vi "Send Single TCP-IP Cmd Abort.vi"(0 "TCP/IP ID":refnum<k5>, 1 "Buffer/Avg #/Frames":u16, 2 "Mode":u16, 3 "Exposure Time (ms)":u32, 4 "Camera Color":string(combo), 5 "Error In":errorcluster, 6 "Function #":u16, 7 "File Name":string, 9 "Parameter Value":i32, 10 "Camera ID":u8=1, 11 "Save As":u16(ring) items=["U16 FITS", "I16 FITS", "I32 FITS", "SGL FITS", "U16 TIFF", "I16 TIFF", "I32 TIFF", "SGL TIFF"], 12 "Acq. Mode/Type/Frame Mode/RO Mode #":u8, 13 "CCD Format Parameters":T1={"Serial Origin"=50, "Serial Length"=512, "Serial Binning"=1, "Parallel Origin"=0, "Parallel Length"=1024, "Parallel Binning"=1} {"Parallel Binning" min=1 max=5000 step=1; "Parallel Length" min=0 max=65535 step=1; "Parallel Origin" min=0 max=9000 step=1; "Serial Binning" min=1 max=5000 step=1; "Serial Length" min=0 max=65535 step=1; "Serial Origin" min=0 max=9000 step=1}) -> (14 "TCP/IP ID Out":refnum<k5>, 15 "Cmd Packet":string, 17 "Data Type":i32, 18 "Packet ID":i32, 19 "Error Out":errorcluster)   [LabVIEW 2015]
uses:
  Systems/SIcamera_Control/SI_Client_Subvis/CCD Format.ctl
panel:
  # "Parallel"
  # "Serial"
  # "Origin"
  # "Length"
  # "Binning"
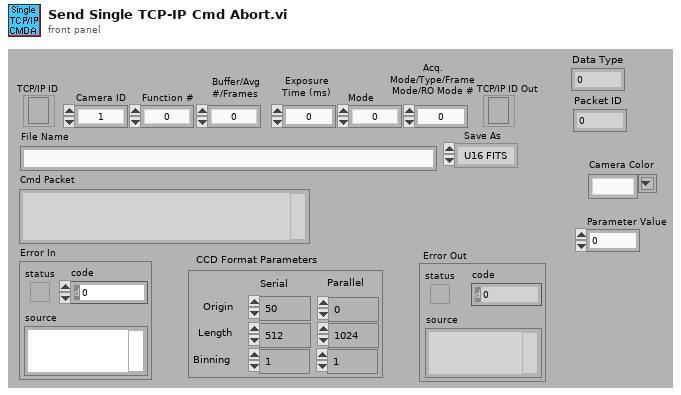
[diagram p1: front panel]
types:
  T1 = typedef "CCD Format.ctl" = cluster{"Serial Origin":i32, "Serial Length":i32, "Serial Binning":i32, "Parallel Origin":i32, "Parallel Length":i32, "Parallel Binning":i32}
  T2 = cluster{"% Exp.":u16, "%Readout":u16, "Relative Pos.":u32, "Acquiring":i32}
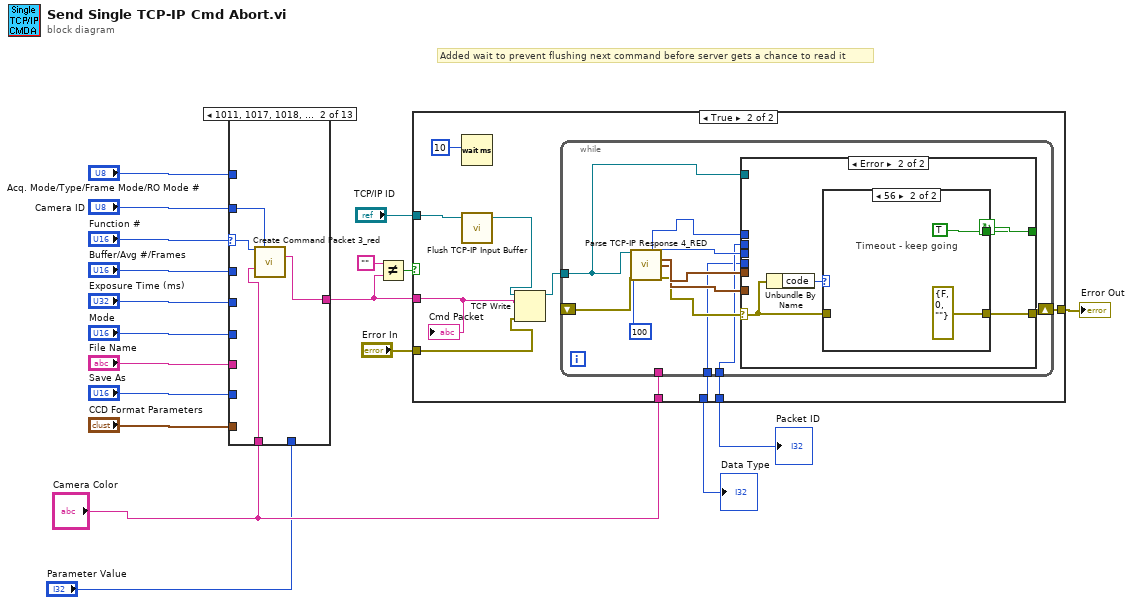
[diagram p0: block diagram]
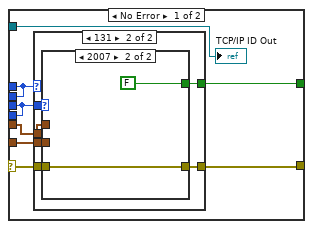
[diagram p3: hidden frame]
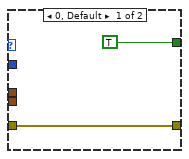
[diagram p4: hidden frame]
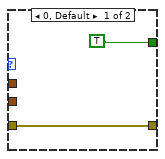
[diagram p5: hidden frame]
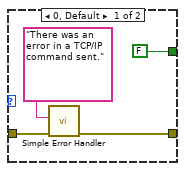
[diagram p6: hidden frame]
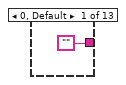
[diagram p7: hidden frame]
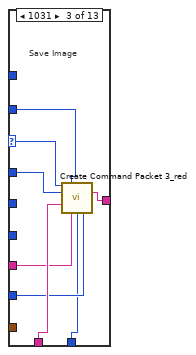
[diagram p8: hidden frame]
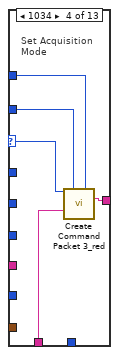
[diagram p9: hidden frame]
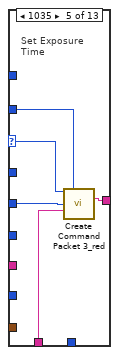
[diagram p10: hidden frame]
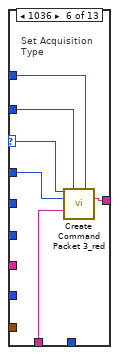
[diagram p11: hidden frame]
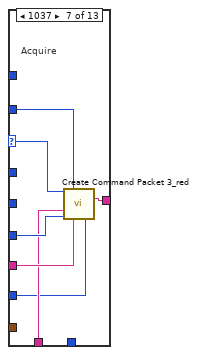
[diagram p12: hidden frame]
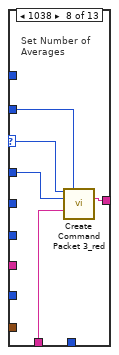
[diagram p13: hidden frame]
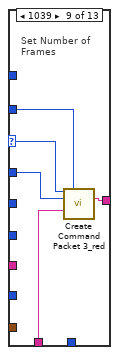
[diagram p14: hidden frame]
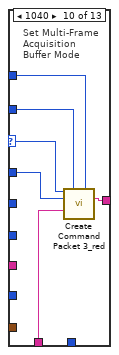
[diagram p15: hidden frame]
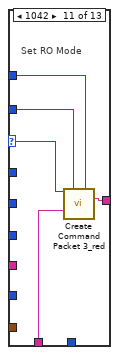
[diagram p16: hidden frame]
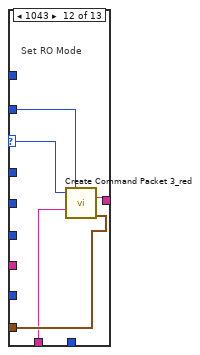
[diagram p17: hidden frame]
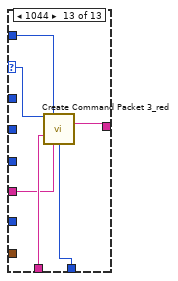
[diagram p18: hidden frame]
diagram:
  # "Added wait to prevent flushing next command before server gets a chance to read it"
  n1 = case shown="1011, 1017, 1018, 1041" "Function #" {
    selector: "Function #" -> [_ w22 w30 w35 w40 w46 w53 w58 w63 w69 w74 w80 w82]
    tunnel: ["" w24 w26 w37 w42 w48 w55 w60 w65 w71 w76 w81 w87] -> w10
    tunnel: "Acq. Mode/Type/Frame Mode/RO Mode #" -> [_ _ _ w34 _ w45 _ _ _ w67 w73 _ _]
    tunnel: "Camera ID" -> [_ w23 w31 w36 w41 w47 w54 w59 w64 w70 w75 w79 w83]
    tunnel: "Buffer/Avg #/Frames" -> [_ _ w29 _ _ w44 _ w57 w62 w68 _ _ _]
    tunnel: "Exposure Time (ms)" -> [_ _ _ _ w39 _ _ _ _ _ _ _ _]
    tunnel: "Mode" -> [_ _ _ _ _ _ w51 _ _ _ _ _ _]
    tunnel: "File Name" -> [_ _ w28 _ _ _ w52 _ _ _ _ _ w84]
    tunnel: "Save As" -> [_ _ w27 _ _ _ w49 _ _ _ _ _ _]
    tunnel: "CCD Format Parameters" -> [_ _ _ _ _ _ _ _ _ _ _ w78 _]
    tunnel: "Camera Color" -> [_ w21 w32 w33 w38 w43 w50 w56 w61 w66 w72 w77 w86]
    tunnel: "Parameter Value" -> [_ _ w25 _ _ _ _ _ _ _ _ _ w85]
    frame 0, Default {
    }
    frame 1011, 1017, 1018, 1041 {
      n2 = call "Create Command Packet 3_red.vi"("Function #"=w22, "Camera ID (1)"=w23, "Camera Color"=w21) -> ("Cmd Packet"=w24:string)  [unwired: 12 in]
    }
    frame 1031 {
      # "Save Image"
      n3 = call "Create Command Packet 3_red.vi"("Function #"=w30, "Camera ID (1)"=w31, "Buffer/Avg #/Frames"=w29, "Camera Color"=w32, "File Name"=w28, "Paramater value"=w25, "Save As"=w27) -> ("Cmd Packet"=w26:string)  [unwired: 8 in]
    }
    frame 1034 {
      # "Set Acquisition Mode"
      n4 = call "Create Command Packet 3_red.vi"("Function #"=w35, "Camera ID (1)"=w36, "Acq. Mode/Type/Frame Mode/RO Mode"=w34, "Camera Color"=w33) -> ("Cmd Packet"=w37:string)  [unwired: 11 in]
    }
    frame 1035 {
      # "Set Exposure Time"
      n5 = call "Create Command Packet 3_red.vi"("Function #"=w40, "Camera ID (1)"=w41, "Exposure Time (ms)"=w39, "Camera Color"=w38) -> ("Cmd Packet"=w42:string)  [unwired: 11 in]
    }
    frame 1036 {
      # "Set Acquisition Type"
      n6 = call "Create Command Packet 3_red.vi"("Function #"=w46, "Camera ID (1)"=w47, "Acq. Mode/Type/Frame Mode/RO Mode"=w45, "Buffer/Avg #/Frames"=w44, "Camera Color"=w43) -> ("Cmd Packet"=w48:string)  [unwired: 10 in]
    }
    frame 1037 {
      # "Acquire"
      n7 = call "Create Command Packet 3_red.vi"("Function #"=w53, "Camera ID (1)"=w54, "Camera Color"=w50, "Mode"=w51, "File Name"=w52, "Save As"=w49) -> ("Cmd Packet"=w55:string)  [unwired: 9 in]
    }
    frame 1038 {
      # "Set Number of Averages"
      n8 = call "Create Command Packet 3_red.vi"("Function #"=w58, "Camera ID (1)"=w59, "Buffer/Avg #/Frames"=w57, "Camera Color"=w56) -> ("Cmd Packet"=w60:string)  [unwired: 11 in]
    }
    frame 1039 {
      # "Set Number of Frames"
      n9 = call "Create Command Packet 3_red.vi"("Function #"=w63, "Camera ID (1)"=w64, "Buffer/Avg #/Frames"=w62, "Camera Color"=w61) -> ("Cmd Packet"=w65:string)  [unwired: 11 in]
    }
    frame 1040 {
      # "Set Multi-Frame Acquisition Buffer Mode"
      n10 = call "Create Command Packet 3_red.vi"("Function #"=w69, "Camera ID (1)"=w70, "Acq. Mode/Type/Frame Mode/RO Mode"=w67, "Buffer/Avg #/Frames"=w68, "Camera Color"=w66) -> ("Cmd Packet"=w71:string)  [unwired: 10 in]
    }
    frame 1042 {
      # "Set RO Mode"
      n11 = call "Create Command Packet 3_red.vi"("Function #"=w74, "Camera ID (1)"=w75, "Acq. Mode/Type/Frame Mode/RO Mode"=w73, "Camera Color"=w72) -> ("Cmd Packet"=w76:string)  [unwired: 11 in]
    }
    frame 1043 {
      # "Set RO Mode"
      n12 = call "Create Command Packet 3_red.vi"("Function #"=w80, "Camera ID (1)"=w79, "Camera Color"=w77, "CCD Format Parameters"=w78) -> ("Cmd Packet"=w81:string)  [unwired: 11 in]
    }
    frame 1044 {
      n13 = call "Create Command Packet 3_red.vi"("Function #"=w82, "Camera ID (1)"=w83, "Camera Color"=w86, "File Name"=w84, "Paramater value"=w85) -> ("Cmd Packet"=w87:string)  [unwired: 10 in]
    }
  }
  n14 = Not Equal?(x="", y=w10) -> (x != y?=w11:bool)
  n15 = case shown="True" w11 {
    tunnel: w10 -> [_ w93]
    tunnel: "TCP/IP ID" -> [_ w98]
    tunnel: "Error In" -> [w88 w94]
    tunnel: [w88 w97] -> w7
    tunnel: "Camera Color" -> [_ w96]
    tunnel: [_ w90] -> w2
    tunnel: [_ w89] -> w1
    frame False {
    }
    frame True {
      n16 = Wait (ms)(milliseconds to wait=u32 10) -> ()  [unwired: 1 out]
      n17 = call "Flush TCP-IP Input Buffer.vi"("TCP/IP ID"=w98) -> ("TCP/IP ID Out"=w92:refnum<k5>)  [unwired: 4 in]
      n18 = TCP Write(connection ID=w92, data in=w93, error in (no error)=w94) -> (connection ID out=w91:refnum<k5>)  [unwired: 1 in, 2 out]
      n19 = while {
        tunnel: w91 -> [w104]
        shift-right: [w105] -> w97
        shift-left: _ -> [w106]
        tunnel: w96 -> [_]
        tunnel: [w100] -> w90
        tunnel: [w99] -> w89
        stop <- w107 continue-if-true
        n20 = call "Parse TCP-IP Response 4_RED.vi"("TCP/IP ID"=w104, "timeout ms (5000)"=100, "error in (no error)"=w106) -> ("Packet ID"=w102:u8, "Data Type"=w101:u16, "Command Done"=w110:cluster{"Function #":u16}, "Acq. Status"=w109:T2, "error out"=w108:errorcluster)  [unwired: 2 in, 6 out]
        n21 = case shown="Error" w108 {
          selector: w108 -> [w115 w132]
          tunnel: w102 -> [w112 _]
          tunnel: w110 -> [w118 _]
          tunnel: w109 -> [w117 _]
          tunnel: [w116 w134] -> w107
          tunnel: w101 -> [w111 _]
          tunnel: [w114 w131] -> w105
          tunnel: w104 -> [w113 _]
          tunnel: [w112 _] -> w100
          tunnel: [w111 _] -> w99
          frame No Error {
            n22 = case shown="131" w112 {
              tunnel: w118 -> [_ w121]
              tunnel: w117 -> [_ w126]
              tunnel: [TRUE w125] -> w116
              tunnel: w111 -> [_ w124]
              tunnel: w115 -> [w119 w123]
              tunnel: [w119 w122] -> w114
              frame 0, Default {
              }
              frame 131 {
                n23 = case shown="2007" w124 {
                  tunnel: w126 -> [_ _]
                  tunnel: [TRUE FALSE] -> w125
                  tunnel: [w127 w129] -> w122
                  tunnel: w123 -> [w127 w129]
                  tunnel: w121 -> [_ _]
                  frame 0, Default {
                  }
                  frame 2007 {
                  }
                }
              }
            }
            "TCP/IP ID Out" <- w113
          }
          frame Error {
            n24 = Unbundle By Name(w132) -> ("code"=w133:i32)
            n25 = case shown="56" w133 {
              tunnel: w132 -> [w138 _]
              tunnel: [FALSE TRUE] -> w134
              tunnel: [w135 errorcluster {"status"=FALSE, "code"=0, "source"=""} ("error out")] -> w131
              frame 0, Default {
                n26 = call <vilib>:"Simple Error Handler.vi"("error source (\" \")"="There was an error in a TCP/IP command sent.", "error in (no error)"=w138) -> ("error out"=w135:errorcluster)  [unwired: 3 in, 4 out]
              }
              frame 56 {
                # "Timeout - keep going"
              }
            }
          }
        }
      }
      "Cmd Packet" <- w93
    }
  }
  "Error Out" <- w7
  "Data Type" <- w1
  "Packet ID" <- w2
